vi "Select init.vi"(8 "error in (no error)":errorcluster, 11 "output cluster":T1) -> (0 "error out":errorcluster)   [LabVIEW 2015, in "ZenGage v3.0 UI.lvclass"]
uses:
  ZenGage v3.0 UI.lvclass
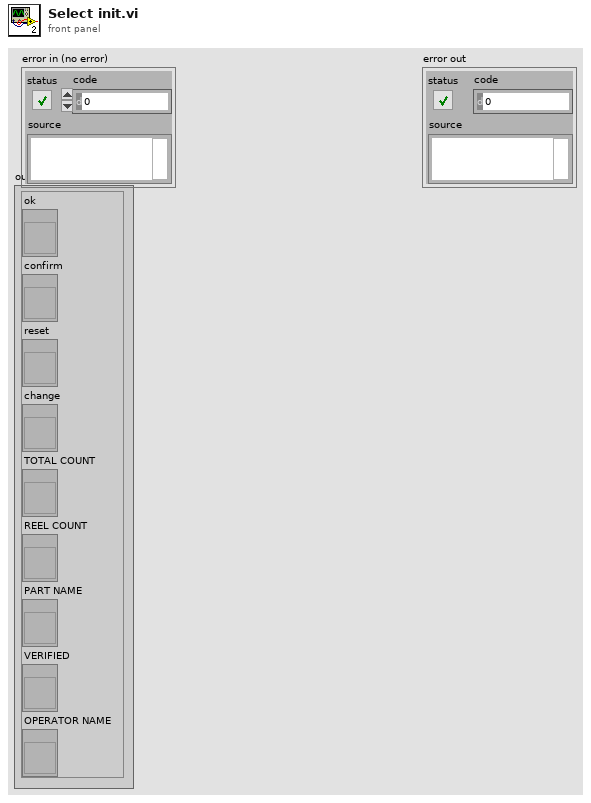
[diagram p1: front panel]
types:
  T1 = cluster{"ok":refnum<vi>, "confirm":refnum<vi>, "reset":refnum<vi>, "change":refnum<vi>, "TOTAL COUNT":refnum<vi>, "REEL COUNT":refnum<vi>, "PART NAME":refnum<vi>, "VERIFIED":refnum<vi>, "OPERATOR NAME":refnum<vi>}
  T2 = enum8{"Enabled", "Disabled", "Disabled and Grayed Out"}
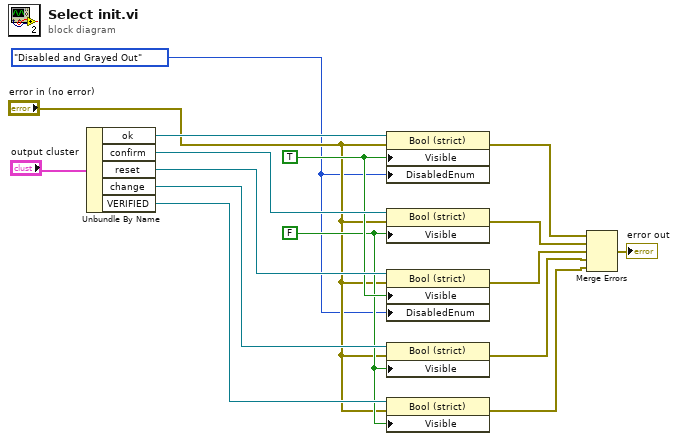
[diagram p0: block diagram]
diagram:
  w1 = T2."Disabled and Grayed Out" ("Disabled")
  w9 = FALSE ("Visible")
  w10 = TRUE ("Visible")
  n1 = Unbundle By Name("output cluster") -> ("ok"=w15:refnum<vi>, "confirm"=w14:refnum<vi>, "reset"=w13:refnum<vi>, "change"=w12:refnum<vi>, "VERIFIED"=w11:refnum<vi>)
  n2 = property class="Bool (strict)"(reference=w15, error in="error in (no error)", "Visible"=w10, "DisabledEnum"=w1) -> (error out=w7:errorcluster)  [unwired: 1 out]
  n3 = property class="Bool (strict)"(reference=w14, error in="error in (no error)", "Visible"=w9) -> (error out=w6:errorcluster)  [unwired: 1 out]
  n4 = property class="Bool (strict)"(reference=w13, error in="error in (no error)", "Visible"=w10, "DisabledEnum"=w1) -> (error out=w5:errorcluster)  [unwired: 1 out]
  n5 = property class="Bool (strict)"(reference=w12, error in="error in (no error)", "Visible"=w9) -> (error out=w4:errorcluster)  [unwired: 1 out]
  n6 = property class="Bool (strict)"(reference=w11, error in="error in (no error)", "Visible"=w9) -> (error out=w3:errorcluster)  [unwired: 1 out]
  n7 = Merge Errors(w7, w6, w5, w4, w3) -> (→"error out":errorcluster)
